vi "Edit User.vi"(4 "Sequence Context":T1) -> (0 "error out":errorcluster)   [LabVIEW 2025]
uses:
  <vilib>/addons/TestStand/_TSLegacy.llb/LabVIEW Test - Sequence Context.ctl
panel:
  in  "LoginName to Edit":string
  in  "OK":bool
  in  "Cancel":bool
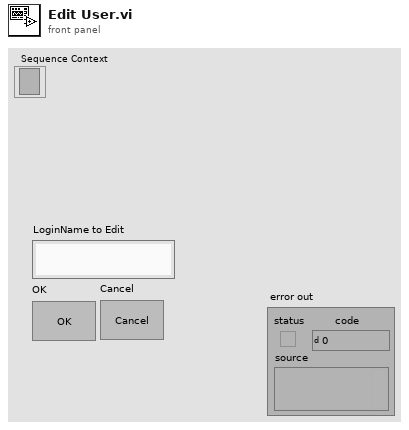
[diagram p1: front panel]
types:
  T1 = typedef "LabVIEW Test - Sequence Context.ctl" = refnum<k7>
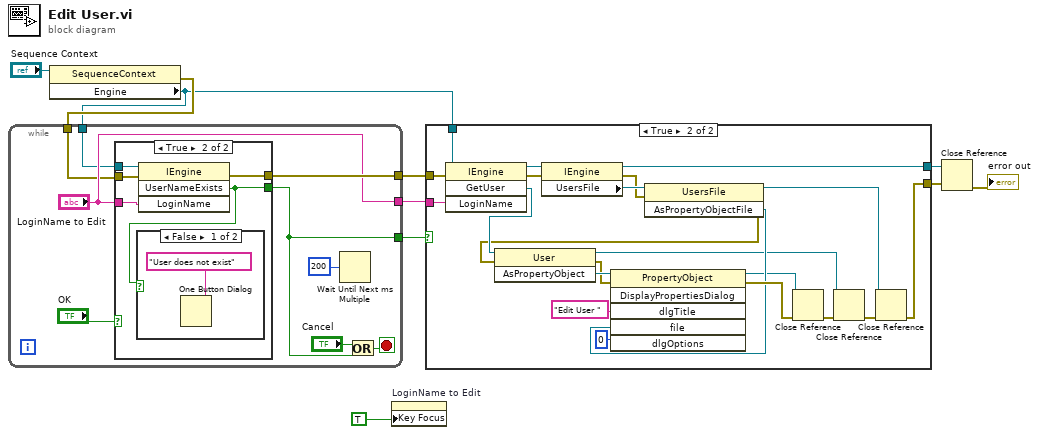
[diagram p0: block diagram]
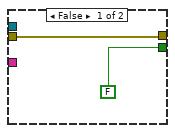
[diagram p2: hidden frame]
diagram:
  n1 = property class="SequenceContext"(reference="Sequence Context") -> (error out=w3:errorcluster, "Engine"=w2:refnum<k7>)  [unwired: 1 in, 1 out]
  n2 = while {
    tunnel: [w11] -> w1
    tunnel: w2 -> [w12]
    tunnel: w3 -> [w13]
    tunnel: ["LoginName to Edit"] -> w4
    tunnel: [w15] -> w10
    stop <- w17 stop-if-true
    n3 = case shown="True" "OK" {
      tunnel: w12 -> [_ w26]
      tunnel: w13 -> [w20 w24]
      tunnel: [w20 w25] -> w15
      tunnel: "LoginName to Edit" -> [_ w23]
      tunnel: [FALSE w22] -> w11
      frame False {
      }
      frame True {
        n4 = invoke class="IEngine" method="UserNameExists"(reference=w26, error in=w24, "LoginName"=w23) -> (error out=w25:errorcluster, "UserNameExists"=w22:bool)  [unwired: 1 in, 2 out]
        n5 = case shown="False" w22 {
          frame False {
            n6 = One Button Dialog(message="User does not exist") -> ()  [unwired: 1 in, 1 out]
          }
          frame True {
          }
        }
      }
    }
    n7 = Wait Until Next ms Multiple(millisecond multiple=u32 200) -> ()  [unwired: 1 out]
    n8 = Or(x="Cancel", y=w11) -> (x .or. y?=w17:bool)
  }
  n9 = property on="LoginName to Edit" class="Str"("Key Focus"=TRUE) -> ()  [unwired: 2 in, 2 out]
  n10 = case shown="True" w1 {
    tunnel: [w28 w35] -> w7
    tunnel: [w29 w44] -> w8
    tunnel: w2 -> [w29 w50]
    tunnel: w10 -> [w28 w51]
    tunnel: w4 -> [_ w49]
    frame False {
    }
    frame True {
      n11 = invoke class="IEngine" method="GetUser"(reference=w50, error in=w51, "LoginName"=w49) -> (reference out=w47:refnum<k7>, error out=w48:errorcluster, "GetUser"=w43:refnum<k7>)  [unwired: 1 in, 1 out]
      n12 = property class="IEngine"(reference=w47, error in=w48) -> (reference out=w44:refnum<k7>, error out=w45:errorcluster, "UsersFile"=w46:refnum<k7>)
      n13 = invoke class="UsersFile" method="AsPropertyObjectFile"(reference=w46, error in=w45) -> (reference out=w31:refnum<k7>, error out=w30:errorcluster, "AsPropertyObjectFile"=w34:refnum<k7>)  [unwired: 1 in]
      n14 = invoke class="User" method="AsPropertyObject"(reference=w43, error in=w30) -> (reference out=w32:refnum<k7>, error out=w41:errorcluster, "AsPropertyObject"=w42:refnum<k7>)  [unwired: 1 in]
      n15 = invoke class="PropertyObject" method="DisplayPropertiesDialog"(reference=w42, error in=w41, "dlgTitle"="Edit User ", "file"=w34, "dlgOptions"=0) -> (reference out=w33:refnum<k7>, error out=w38:errorcluster)  [unwired: 1 in, 4 out]
      n16 = Close Reference(reference=w33, error in (no error)=w38) -> (error out=w37:errorcluster)
      n17 = Close Reference(reference=w32, error in (no error)=w37) -> (error out=w36:errorcluster)
      n18 = Close Reference(reference=w31, error in (no error)=w36) -> (error out=w35:errorcluster)
    }
  }
  n19 = Close Reference(reference=w8, error in (no error)=w7) -> (error out=→"error out":errorcluster)
